vi "Post Build Script.vi"(8 "error in (no error)":errorcluster, 11 "PostBuildSupport in":refnum<class "PostBuildSupport.lvclass">) -> (0 "error out":errorcluster)   [LabVIEW 2016, in "PostBuildSupport.lvclass"]
uses:
  PostBuildSupport.lvclass
  <vilib>/addons/WireFlow/_WF_ProgressBar.llb/ProgressBar_WireFlow.lvclass
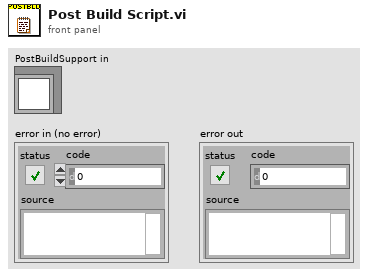
[diagram p1: front panel]
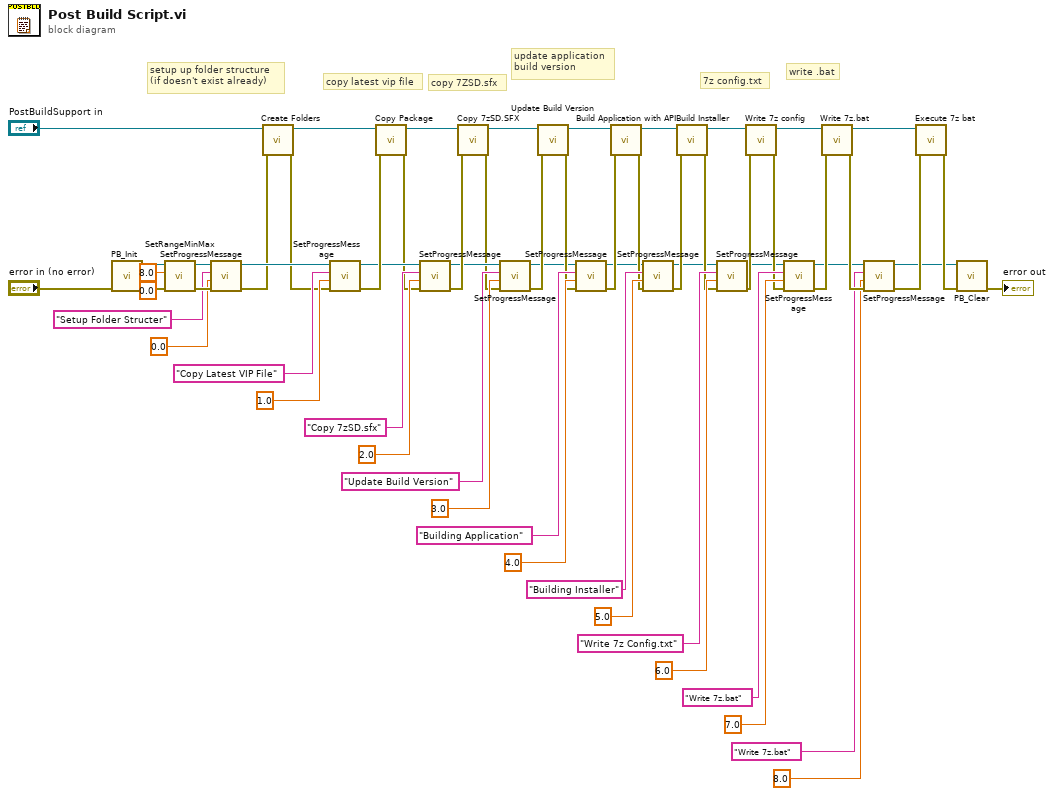
[diagram p0: block diagram]
diagram:
  # "copy 7ZSD.sfx"
  # "setup up folder structure \n(if doesn't exist already)"
  # "update application\nbuild version"
  # "copy latest vip file"
  # "7z config.txt"
  # "write .bat"
  n1 = call <vilib>:"PB_Init.vi"("error in (no error)"="error in (no error)") -> ("error out"=w53:errorcluster, "WF-ProgressBar out"=w17:refnum<class "ProgressBar_WireFlow.lvclass">)  [unwired: 9 in]
  n2 = call-dynamic "SetRangeMinMax.vi"("error in (no error)"=w53, "Min (0)"=0.0, "Max (1)"=8.0, "WF-ProgressBar in"=w17) -> ("error out"=w51:errorcluster, "WF-ProgressBar out"=w18:refnum<class "ProgressBar_WireFlow.lvclass">)  [unwired: 6 in]
  n3 = call-dynamic "SetProgressMessage.vi"("error in (no error)"=w51, "Progress value (NaN no update)"=0.0, "Message"="Setup Folder Structer", "WF-ProgressBar in"=w18) -> ("error out"=w13:errorcluster, "WF-ProgressBar out"=w25:refnum<class "ProgressBar_WireFlow.lvclass">)  [unwired: 5 in, 1 out]
  n4 = call "Create Folders.vi"("error in (no error)"=w13, "PostBuildSupport in"="PostBuildSupport in") -> ("error out"=w12:errorcluster, "PostBuildSupport out"=w60:refnum<class "PostBuildSupport.lvclass">)  [unwired: 8 in]
  n5 = call-dynamic "SetProgressMessage.vi"("error in (no error)"=w12, "Progress value (NaN no update)"=1.0, "Message"="Copy Latest VIP File", "WF-ProgressBar in"=w25) -> ("error out"=w48:errorcluster, "WF-ProgressBar out"=w16:refnum<class "ProgressBar_WireFlow.lvclass">)  [unwired: 5 in, 1 out]
  n6 = call "Copy Package.vi"("error in (no error)"=w48, "PostBuildSupport in"=w60) -> ("error out"=w15:errorcluster, "PostBuildSupport out"=w59:refnum<class "PostBuildSupport.lvclass">)  [unwired: 8 in]
  n7 = call-dynamic "SetProgressMessage.vi"("error in (no error)"=w15, "Progress value (NaN no update)"=2.0, "Message"="Copy 7zSD.sfx", "WF-ProgressBar in"=w16) -> ("error out"=w34:errorcluster, "WF-ProgressBar out"=w24:refnum<class "ProgressBar_WireFlow.lvclass">)  [unwired: 5 in, 1 out]
  n8 = call "Copy 7zSD.SFX.vi"("error in (no error)"=w34, "PostBuildSupport in"=w59) -> ("error out"=w14:errorcluster, "PostBuildSupport out"=w58:refnum<class "PostBuildSupport.lvclass">)  [unwired: 8 in]
  n9 = call-dynamic "SetProgressMessage.vi"("error in (no error)"=w14, "Progress value (NaN no update)"=3.0, "Message"="Update Build Version", "WF-ProgressBar in"=w24) -> ("error out"=w33:errorcluster, "WF-ProgressBar out"=w23:refnum<class "ProgressBar_WireFlow.lvclass">)  [unwired: 5 in, 1 out]
  n10 = call "Update Build Version.vi"("error in (no error)"=w33, "PostBuildSupport in"=w58) -> ("error out"=w32:errorcluster, "PostBuildSupport out"=w57:refnum<class "PostBuildSupport.lvclass">)  [unwired: 8 in]
  n11 = call-dynamic "SetProgressMessage.vi"("error in (no error)"=w32, "Progress value (NaN no update)"=4.0, "Message"="Building Application", "WF-ProgressBar in"=w23) -> ("error out"=w31:errorcluster, "WF-ProgressBar out"=w22:refnum<class "ProgressBar_WireFlow.lvclass">)  [unwired: 5 in, 1 out]
  n12 = call "Build Application with API.vi"("error in (no error)"=w31, "PostBuildSupport in"=w57) -> ("error out"=w30:errorcluster, "PostBuildSupport out"=w55:refnum<class "PostBuildSupport.lvclass">)  [unwired: 8 in]
  n13 = call-dynamic "SetProgressMessage.vi"("error in (no error)"=w30, "Progress value (NaN no update)"=5.0, "Message"="Building Installer", "WF-ProgressBar in"=w22) -> ("error out"=w29:errorcluster, "WF-ProgressBar out"=w21:refnum<class "ProgressBar_WireFlow.lvclass">)  [unwired: 5 in, 1 out]
  n14 = call "Build Installer.vi"("error in (no error)"=w29, "PostBuildSupport in"=w55) -> ("error out"=w28:errorcluster, "PostBuildSupport out"=w56:refnum<class "PostBuildSupport.lvclass">)  [unwired: 8 in]
  n15 = call-dynamic "SetProgressMessage.vi"("error in (no error)"=w28, "Progress value (NaN no update)"=6.0, "Message"="Write 7z Config.txt", "WF-ProgressBar in"=w21) -> ("error out"=w27:errorcluster, "WF-ProgressBar out"=w20:refnum<class "ProgressBar_WireFlow.lvclass">)  [unwired: 5 in, 1 out]
  n16 = call "Write 7z config.vi"("error in (no error)"=w27, "PostBuildSupport in"=w56) -> ("error out"=w26:errorcluster, "PostBuildSupport out"=w61:refnum<class "PostBuildSupport.lvclass">)  [unwired: 8 in]
  n17 = call-dynamic "SetProgressMessage.vi"("error in (no error)"=w26, "Progress value (NaN no update)"=7.0, "Message"="Write 7z.bat", "WF-ProgressBar in"=w20) -> ("error out"=w19:errorcluster, "WF-ProgressBar out"=w8:refnum<class "ProgressBar_WireFlow.lvclass">)  [unwired: 5 in, 1 out]
  n18 = call "Write 7z.bat.vi"("error in (no error)"=w19, "PostBuildSupport in"=w61) -> ("error out"=w9:errorcluster, "PostBuildSupport out"=w6:refnum<class "PostBuildSupport.lvclass">)  [unwired: 8 in]
  n19 = call-dynamic "SetProgressMessage.vi"("error in (no error)"=w9, "Progress value (NaN no update)"=8.0, "Message"="Write 7z.bat", "WF-ProgressBar in"=w8) -> ("error out"=w7:errorcluster, "WF-ProgressBar out"=w2:refnum<class "ProgressBar_WireFlow.lvclass">)  [unwired: 5 in, 1 out]
  n20 = call "Execute 7z bat.vi"("error in (no error)"=w7, "PostBuildSupport in"=w6) -> ("error out"=w3:errorcluster)  [unwired: 8 in, 1 out]
  n21 = call-dynamic "PB_Clear.vi"("error in (no error)"=w3, "WF-ProgressBar in"=w2) -> ("error out"=→"error out":errorcluster)  [unwired: 8 in, 1 out]
